vi "Write Enums As String.vi"(10 "Enums As String (F)":bool, 11 "Serializer.JSON in":refnum<class "Serializer.JSON.lvclass">) -> (3 "Serializer.JSON out":refnum<class "Serializer.JSON.lvclass">)   [LabVIEW 2013, in "OpenSerializer.JKI-JSON.lvlib" / "Serializer.JSON.lvclass"]
uses:
  Serializer.JSON.lvclass
  Serializer.JSON.lvclass/Serializer.JSON.ctl
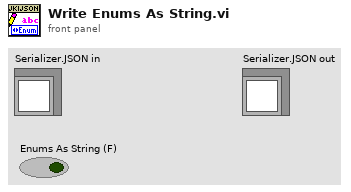
[diagram p1: front panel]
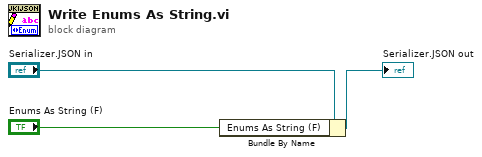
[diagram p0: block diagram]
diagram:
  n1 = Bundle By Name(cluster="Serializer.JSON in", "Enums As String (F)"="Enums As String (F)") -> (→"Serializer.JSON out":refnum<class "Serializer.JSON.lvclass">)
